vi "Main Loop.vi"(8 "error in (no error)":errorcluster, 10 "Init options":T1={"List"=[], "max rows"=8, "Listbox placement"=enum."None", "String Color Options"={"Use? (F)"=FALSE, "Color - Valid"=0, "Color - Invalid"=0, "Allow blank?"=FALSE}}, 11 "Handle":refnum<class "Handle.lvclass">) -> (0 "error out":errorcluster, 2 "Ref.Listbox":refnum<vi>, 3 "Ref.String":refnum<vi>)   [LabVIEW 2021, in "Autocomplete Textbox.lvlib" / "Handle.lvclass"]
uses:
  Classes/Handle/Handle.lvclass
  Classes/Handle/Init inputs.ctl
  Classes/Handle/Listbox placement.ctl
  SubVIs/Color String Options.ctl
  SubVIs/Loop Data.ctl
  SubVIs/Inputs.ctl
  SubVIs/Refs.ctl
  SubVIs/State data.ctl
  Classes/Handle/Handle.lvclass/Handle.ctl
  <userlib>/_OpenG.lib/array/array.llb/Remove Duplicates from 1D Array__ogtk.vi
  <userlib>/_OpenG.lib/array/array.llb/Remove Duplicates from 1D Array (String)__ogtk.vi
  <userlib>/_OpenG.lib/array/array.llb/Filter 1D Array__ogtk.vi
  <userlib>/_OpenG.lib/array/array.llb/Filter 1D Array with Scalar (String)__ogtk.vi
  Autocomplete Textbox.lvlib
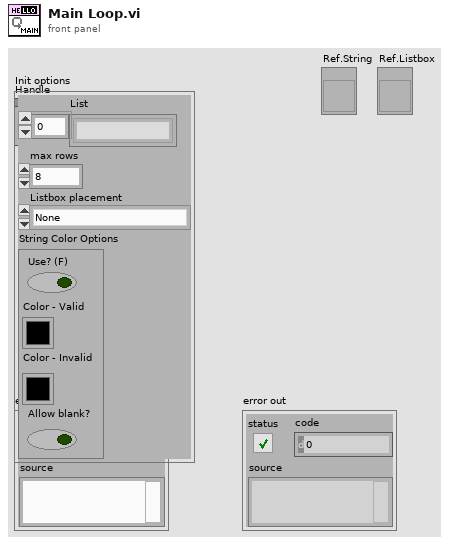
[diagram p1: front panel]
types:
  T1 = typedef "Autocomplete Textbox.lvlib/Handle.lvclass/Init inputs.ctl" = cluster{"List":string[], "max rows":i32, "Listbox placement":T2, "String Color Options":T3}
  T2 = typedef "Autocomplete Textbox.lvlib/Handle.lvclass/Listbox placement.ctl" = enum16{"None", "Under String", "Fit to Pane"}
  T3 = typedef "Autocomplete Textbox.lvlib/Color String Options.ctl" = cluster{"Use? (F)":bool, "Color - Valid":u32, "Color - Invalid":u32, "Allow blank?":bool}
  T4 = typedef "Autocomplete Textbox.lvlib/Inputs.ctl" = cluster{"List":string[], "max rows":i32, "Listbox placement":T2, "String Color Options":T3}
  T5 = typedef "Autocomplete Textbox.lvlib/Loop Data.ctl" = cluster{"Config":T4, "Refs":T6, "State":T7}
  T6 = typedef "Autocomplete Textbox.lvlib/Refs.ctl" = cluster{"String":refnum<vi>, "Listbox":refnum<vi>}
  T7 = typedef "Autocomplete Textbox.lvlib/State data.ctl" = cluster{"LB active?":bool}
  T8 = typedef "eventvkey.ctl" = enum16{"ASCII", "Enter", "Return", "Shift", "Ctrl", "Alt", "Cmd", "Opt", "Caps", "NumLock", "Clear", "Break", "Up", "Down", "Left", "Right", "Insert", "Delete", "Home", "End", "PageUp", "PageDown", "Escape", "Help", "Pause", "ScrollLock", "F1", "F2", "F3", "F4", "F5", "F6", "F7", "F8", "F9", "F10", "F11", "F12", "F13", "F14", "F15", "F16", "F17", "F18", "F19", "F20", "F21", "F22", "F23", "F24", "Play", "VolumeUp", "VolumeDown", "Mute", "Two Byte Char"}
  T9 = typedef "LVPoint32TypeDef.ctl" = cluster{"Horizontal":i32, "Vertical":i32}
  T10 = typedef "Autocomplete Textbox.lvlib/Handle.lvclass/ToMain UE action.ctl" = enum16{"New List", "Shutdown", "New Value", "Mouse Down (signal)"}
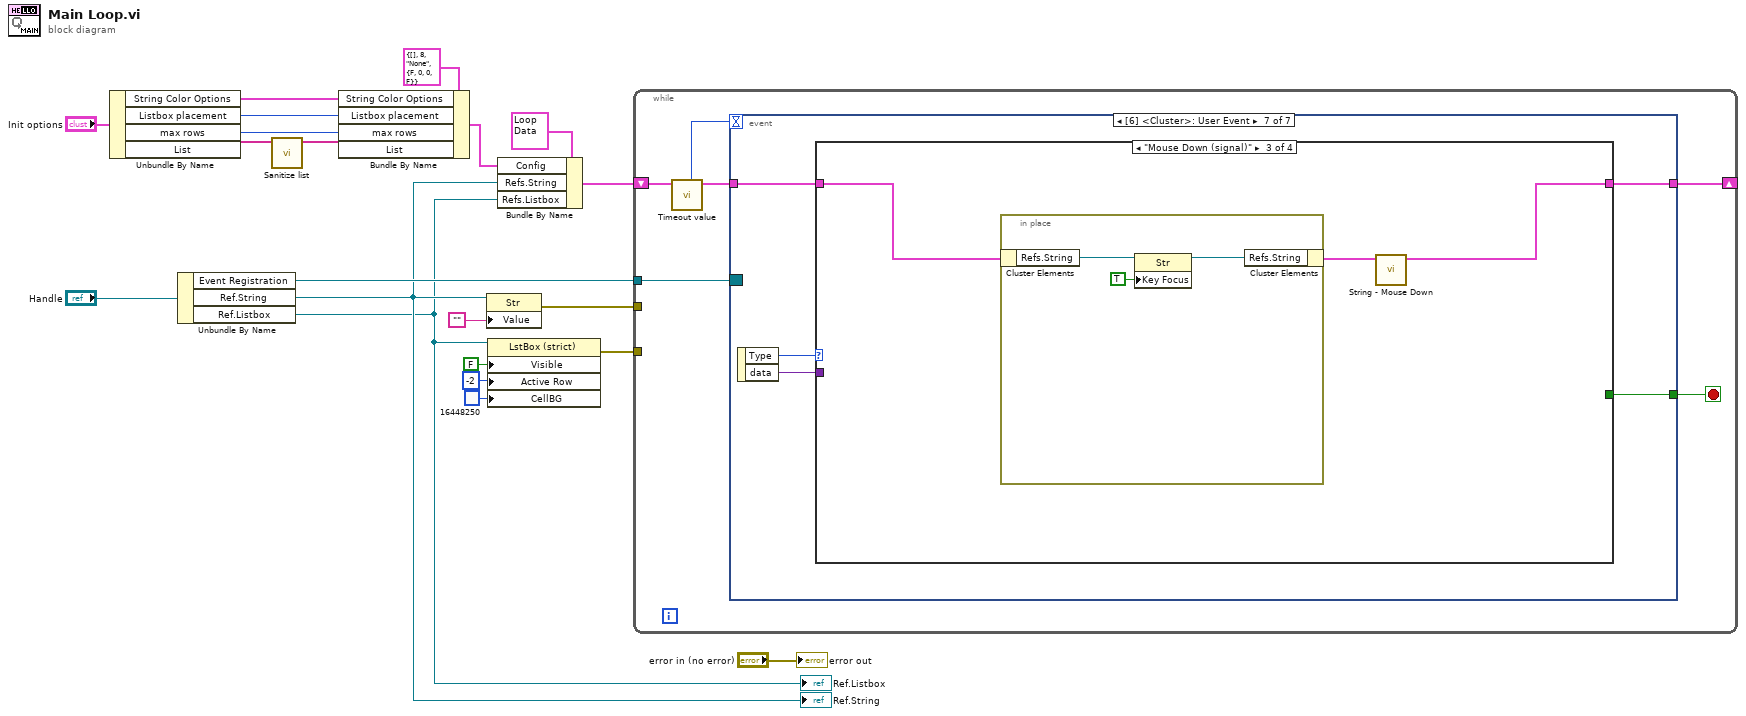
[diagram p0: block diagram]
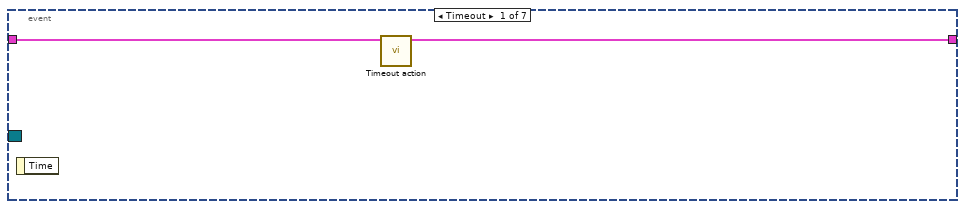
[diagram p2: hidden frame]
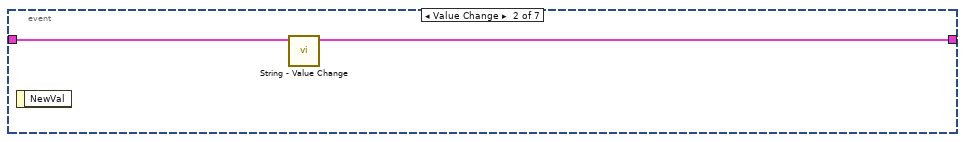
[diagram p3: hidden frame]
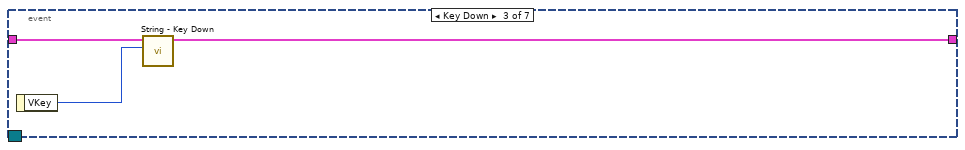
[diagram p4: hidden frame]
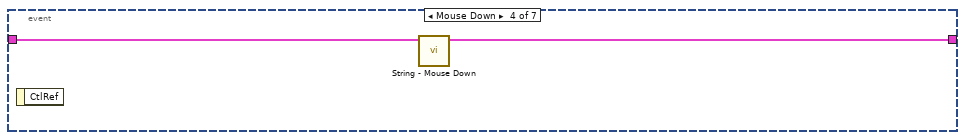
[diagram p5: hidden frame]
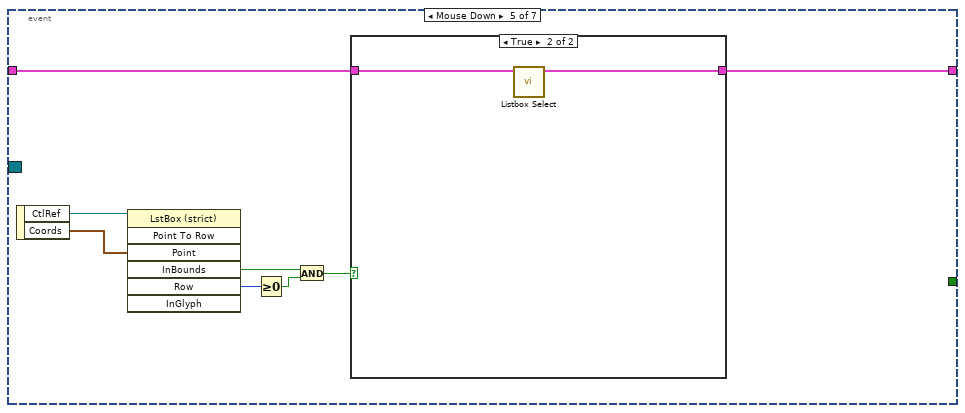
[diagram p6: hidden frame]
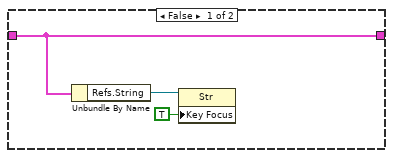
[diagram p7: hidden frame]
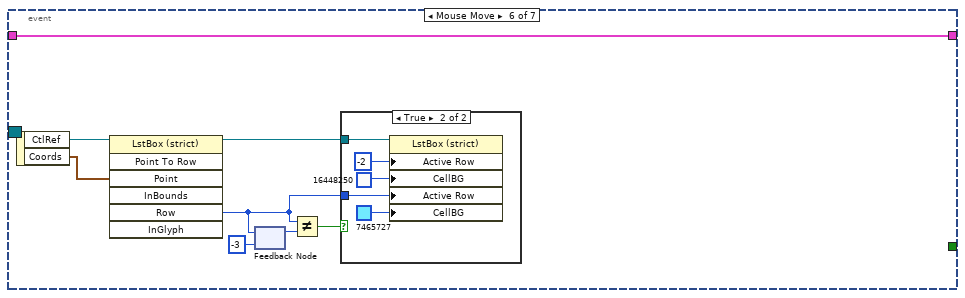
[diagram p8: hidden frame]
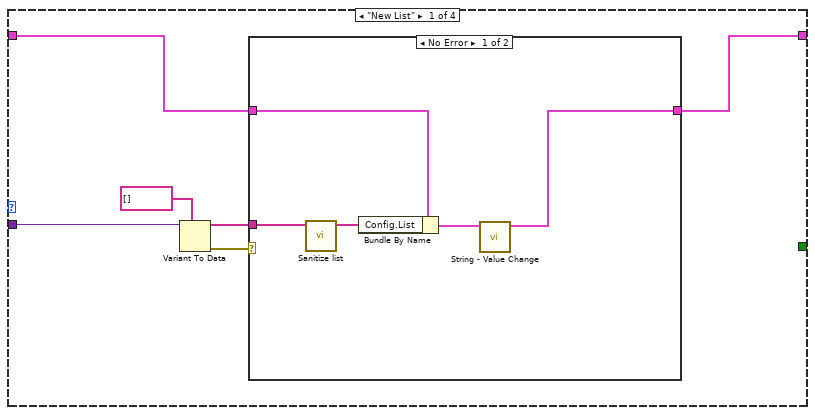
[diagram p10: hidden frame]
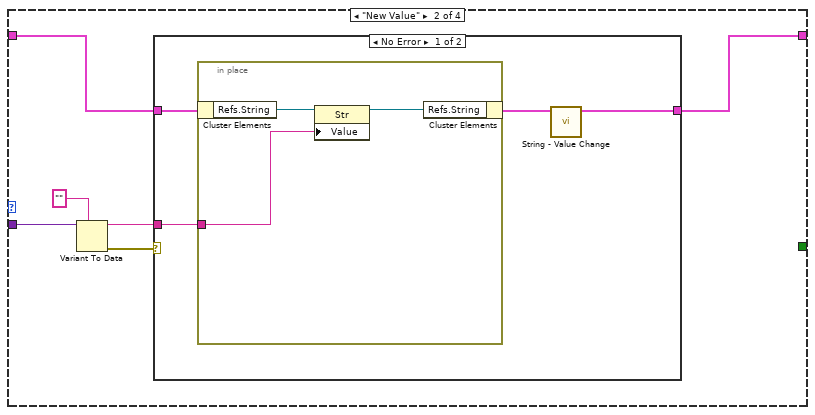
[diagram p12: hidden frame]
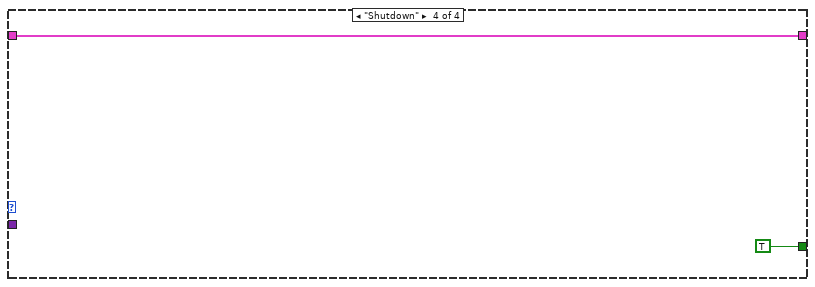
[diagram p14: hidden frame]
diagram:
  n1 = Unbundle By Name("Init options") -> ("String Color Options"=w1:T3, "Listbox placement"=w2:T2, "max rows"=w10:i32, "List"=w4:string[])
  n2 = Unbundle By Name("Handle") -> ("Event Registration"=w8:refnum<event-registration>, "Ref.String"=w7:refnum<vi>, "Ref.Listbox"=w6:refnum<vi>)
  "Ref.String" <- w7
  "Ref.Listbox" <- w6
  n3 = call "Sanitize list.vi"("List"=w4) -> ("sanitized list"=w3:string[])  [unwired: 10 in]
  n4 = Bundle By Name(cluster=T4 {"List"=[], "max rows"=8, "Listbox placement"=enum."None", "String Color Options"={"Use? (F)"=FALSE, "Color - Valid"=0, "Color - Invalid"=0, "Allow blank?"=FALSE}} ("Config"), "String Color Options"=w1, "Listbox placement"=w2, "max rows"=w10, "List"=w3) -> (w18:T4)
  n5 = property class="Str"(reference=w7, "Value"="") -> (error out=w12:errorcluster)  [unwired: 1 in, 1 out]
  n6 = property class="LstBox (strict)"(reference=w6, "Visible"=FALSE, "Active Row"=-2 ("Active Row:Active Row Number"), "CellBG"=u32 16448250) -> (error out=w14:errorcluster)  [unwired: 1 in, 1 out]
  n7 = Bundle By Name(cluster=T5 {"Config"={"List"=[], "max rows"=8, "Listbox placement"=enum."None", "String Color Options"={"Use? (F)"=FALSE, "Color - Valid"=0, "Color - Invalid"=0, "Allow blank?"=FALSE}}, "Refs"={"String"=refnum, "Listbox"=refnum}, "State"={"LB active?"=FALSE}} ("Cluster"), "Config"=w18, "Refs.String"=w7, "Refs.Listbox"=w6) -> (w20:T5)
  n8 = while {
    tunnel: w8 -> [w27]
    shift-right: [w26] -> _
    shift-left: w20 -> [w25]
    tunnel: w14 -> [_]
    tunnel: w12 -> [_]
    stop <- w22 stop-if-true
    n9 = call "Timeout value.vi"("Loop data in"=w25) -> ("Loop data out"=w24:T5, "timeout (ms)"=w23:i32)  [unwired: 9 in]
    n10 = event shown="[6] <Cluster>: User Event" {
      selector: w27 -> [_ _ _ _ _ _ _]
      dyn-events: _ -> [_ _ _ _ _ _ _]
      timeout: w23 -> [_ _ _ _ _ _ _]
      tunnel: w24 -> [w29 w31 w34 w36 w38 w50 w64]
      tunnel: [w28 w30 w33 w35 w37 w50 w63] -> w26
      tunnel: [_ _ _ _ _ _ w65] -> w22
      event Timeout {
        n11 = event-data() -> ()  [unwired: 1 in, 1 out]
        n12 = call "Timeout action.vi"("Loop data in"=w29) -> ("Loop data out"=w28:T5)  [unwired: 9 in, 1 out]
      }
      event Value Change {
        n13 = event-data() -> ()  [unwired: 1 in, 1 out]
        n14 = call "String - Value Change.vi"("Loop data in"=w31) -> ("Loop data out"=w30:T5)  [unwired: 9 in, 1 out]
      }
      event Key Down {
        n15 = event-data() -> ("VKey"=w32:T8)  [unwired: 1 in]
        n16 = call "String - Key Down.vi"("VKey"=w32, "Loop data in"=w34) -> ("Loop data out"=w33:T5)  [unwired: 8 in, 1 out]
      }
      event Mouse Down {
        n17 = event-data() -> ()  [unwired: 1 in, 1 out]
        n18 = call "String - Mouse Down.vi"("Loop data in"=w36) -> ("Loop data out"=w35:T5)  [unwired: 9 in, 1 out]
      }
      event Mouse Down {
        n19 = event-data() -> ("CtlRef"=w44:refnum<vi>, "Coords"=w43:T9)  [unwired: 1 in]
        n20 = invoke class="LstBox (strict)" method="Point To Row"(reference=w44, "Point"=w43) -> ("InBounds"=w41:bool, "Row"=w42:i32)  [unwired: 5 in, 5 out]
        n21 = Greater Or Equal To 0?(x=w42) -> (x >= 0?=w40:bool)
        n22 = And(x=w41, y=w40) -> (x .and. y?=w39:bool)
        n23 = case shown="True" w39 {
          tunnel: w38 -> [w45 w49]
          tunnel: [w45 w48] -> w37
          frame False {
            n24 = Unbundle By Name(w45) -> ("Refs.String"=w46:refnum<vi>)
            n25 = property on="Property Node" class="Str"(reference=w46, "Key Focus"=TRUE) -> ()  [unwired: 1 in, 2 out]
          }
          frame True {
            n26 = call "Listbox Select.vi"("Loop data in"=w49) -> ("Loop data out"=w48:T5)  [unwired: 9 in, 1 out]
          }
        }
      }
      event Mouse Move {
        n27 = event-data() -> ("CtlRef"=w52:refnum<vi>, "Coords"=w51:T9)  [unwired: 1 in]
        n28 = invoke class="LstBox (strict)" method="Point To Row"(reference=w52, "Point"=w51) -> (reference out=w57:refnum<vi>, "Row"=w54:i32)  [unwired: 5 in, 5 out]
        n29 = feedback #1(-3 ("Row")) -> (w55:i32)
        n30 = feedback-in #1(w54) -> ()
        n31 = Not Equal?(x=w54, y=w55) -> (x != y?=w53:bool)
        n32 = case shown="True" w53 {
          tunnel: w57 -> [_ w59]
          tunnel: w54 -> [_ w58]
          frame False {
          }
          frame True {
            n33 = property class="LstBox (strict)"(reference=w59, "Active Row"=-2 ("Active Row:Active Row Number"), "CellBG"=u32 16448250, "Active Row"=w58, "CellBG"=u32 7465727) -> ()  [unwired: 1 in, 2 out]
          }
        }
      }
      event User Event {
        n34 = event-data() -> ("Type"=w67:T10, "data"=w66:variant)  [unwired: 1 in]
        n35 = case shown="\"Mouse Down (signal)\"" w67 {
          tunnel: w66 -> [w73 w85 _ _]
          tunnel: [_ _ _ TRUE] -> w65
          tunnel: w64 -> [w69 w81 w96 w100]
          tunnel: [w68 w80 w95 w100] -> w63
          frame "New List" {
            n36 = Variant To Data(type=string[] [], Variant=w73) -> (data=w71:string[], error out=w70:errorcluster)  [unwired: 1 in]
            n37 = case shown="No Error" w70 {
              tunnel: w71 -> [w77 _]
              tunnel: w69 -> [w78 w79]
              tunnel: [w74 w79] -> w68
              frame No Error {
                n38 = call "Sanitize list.vi"("List"=w77) -> ("sanitized list"=w76:string[])  [unwired: 10 in]
                n39 = Bundle By Name(cluster=w78, "Config.List"=w76) -> (w75:T5)
                n40 = call "String - Value Change.vi"("Loop data in"=w75) -> ("Loop data out"=w74:T5)  [unwired: 9 in, 1 out]
              }
              frame Error {
              }
            }
          }
          frame "New Value" {
            n41 = Variant To Data(type="", Variant=w85) -> (data=w83:string, error out=w82:errorcluster)  [unwired: 1 in]
            n42 = case shown="No Error" w82 {
              tunnel: w83 -> [w87 _]
              tunnel: w81 -> [w88 w93]
              tunnel: [w89 w93] -> w80
              frame No Error {
                n43 = in-place {
                  in-place-border: w87 -> [w90]
                  n44 = in-place-cluster #2(w88) -> ("Refs.String"=w92:refnum<vi>)
                  n45 = property class="Str"(reference=w92, "Value"=w90) -> (reference out=w91:refnum<vi>)  [unwired: 1 in, 1 out]
                  n46 = in-place-cluster #2("Refs.String"=w91) -> (w86:T5)
                }
                n47 = call "String - Value Change.vi"("Loop data in"=w86) -> ("Loop data out"=w89:T5)  [unwired: 9 in, 1 out]
              }
              frame Error {
              }
            }
          }
          frame "Mouse Down (signal)" {
            n48 = in-place {
              n49 = in-place-cluster #3(w96) -> ("Refs.String"=w99:refnum<vi>)
              n50 = property class="Str"(reference=w99, "Key Focus"=TRUE) -> (reference out=w98:refnum<vi>)  [unwired: 1 in, 1 out]
              n51 = in-place-cluster #3("Refs.String"=w98) -> (w94:T5)
            }
            n52 = call "String - Mouse Down.vi"("Loop data in"=w94) -> ("Loop data out"=w95:T5)  [unwired: 9 in, 1 out]
          }
          frame "Shutdown" {
          }
        }
      }
    }
  }
  "error out" <- "error in (no error)"
